vi "Write Raw CMD - Single Device.vi"(0 "Data Out":string, 11 "error in":errorcluster, 12 "Log (T)":bool=TRUE, 13 "Device Idx (0-5)":u32, 14 "FPGA":T1) -> (15 "error out":errorcluster)   [LabVIEW 2017, in "Host SRL.lvlib"]
uses:
  Host SRL.lvlib
  Type Defs/WSVCAP SHL FPGA Enum.ctl
panel:
  out "Socket Mask":u32=1 format="%06x"
  out "Data Out":u8[][](array[numeric]) format="%02x"
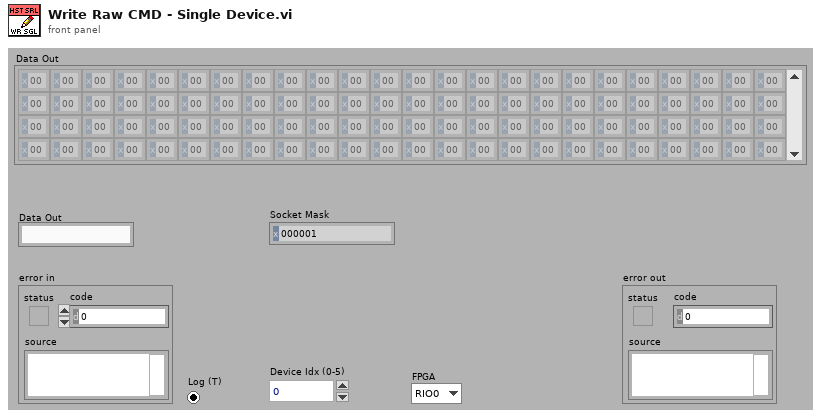
[diagram p1: front panel]
types:
  T1 = typedef "WSVCAP SHL FPGA Enum.ctl" = enum16{"RIO0", "RIO1"}
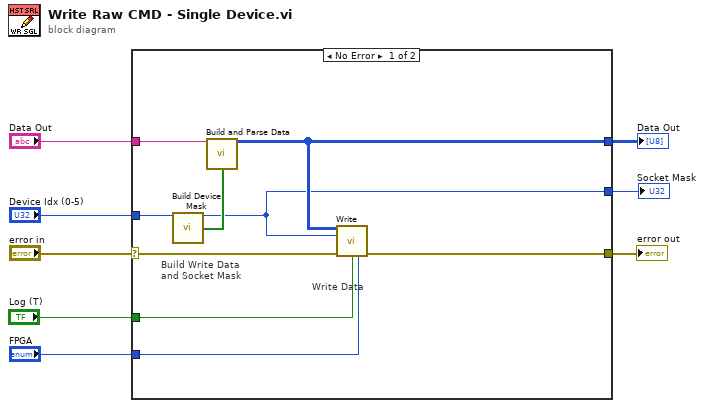
[diagram p0: block diagram]
diagram:
  n1 = case shown="No Error" "error in" {
    selector: "error in" -> [w16 _]
    tunnel: [w15 _] -> w8
    tunnel: "Data Out" -> [w14 _]
    tunnel: [w12 _] -> w5
    tunnel: "Device Idx (0-5)" -> [w17 _]
    tunnel: [w10 _] -> w4
    tunnel: "Log (T)" -> [w11 _]
    tunnel: "FPGA" -> [w9 _]
    frame No Error {
      # "Write Data"
      # "Build Write Data and Socket Mask"
      n2 = call "Build Device Mask.vi"("Device Idx (0-5)"=w17) -> ("Socket Mask [U32]"=w10:u32, "DUT Mask"=w13:bool[])  [unwired: 13 in]
      n3 = call "Build and Parse Data.vi"("SRL Message Out"=w14, "Dev Mask (All)"=w13) -> ("SRL Data Out [U8]"=w12:u8[][])  [unwired: 12 in, 1 out]
      n4 = call "Write.vi"("SRL Data Out"=w12, "Socket Mask"=w10, "error in"=w16, "Log (T)"=w11, "FPGA"=w9) -> ("error out"=w15:errorcluster)  [unwired: 10 in]
    }
    frame Error {
    }
  }
  "error out" <- w8
  "Data Out" <- w5
  "Socket Mask" <- w4
